vi "PH_IEEE1394Camera.get Cam Attributes.vi"(0 "i ref in":refnum<vi>, 2 "IMAQ1394 Session In":T1, 4 "Cam Error in":errorcluster, 5 "error in (no error)":errorcluster) -> (14 "i ref out":refnum<vi>, 16 "IMAQ1394 Session Out":T1, 18 "Cam Error out":errorcluster, 19 "error out":errorcluster)   [LabVIEW 2014, in "PH_IEEE1394Camera.lvlib"]
doc: "This VI gets the cam attributes and sets them to the GUI element."
uses:
  PH_IEEE1394Camera.lvlib
  <vilib>/userdefined/High Color/IMAQdx.ctl
  <vilib>/vision/driver/NI_Vision_Acquisition_Software.lvlib
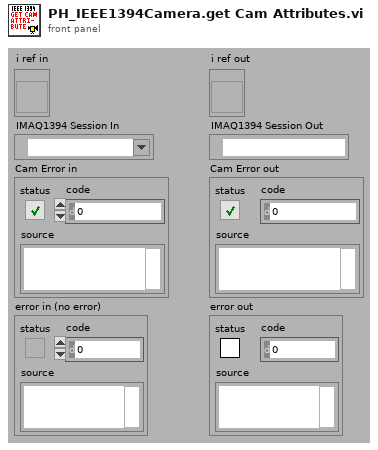
[diagram p1: front panel]
types:
  T1 = typedef "IMAQdx.ctl" = refnum<k21>
  T2 = typedef "PH_IEEE1394Camera.lvlib/PH_IEEE1394Camera.i attribute.ctl" = cluster{"Gui Refs":cluster{"Brightness":refnum<vi>, "Shutter":refnum<vi>, "Gain":refnum<vi>, "Center of Gravity":refnum<vi>, "Supported Video Modes":refnum<vi>, "Trigger Polarity":refnum<vi>, "Trigger Mode":refnum<vi>, "Trigger Timeout":refnum<vi>, "Bit Depth":refnum<vi>, "Video Mode":refnum<vi>, "Top":refnum<vi>, "Bottom":refnum<vi>, "Left":refnum<vi>, "Right":refnum<vi>, "Set ROI to Maximum":refnum<vi>, "Camera Details":refnum<vi>, "Current Cam Attributes":refnum<vi>, "Attribute to set":refnum<vi>, "Num Value":refnum<vi>, "String Value":refnum<vi>, "Bool Value":refnum<vi>, "Set Cam Attribute":refnum<vi>}, "Cam":cluster{"IMAQ1394 Session":T1, "Camera Details":T3}, "Current Attributes":T4[], "Supported Video Modes ":cluster{"Video Mode":u32, "Video Mode Name":string}[], "Wanted Attributes":cluster{"Name":string, "Num Value":dbl, "String Value":string, "Boolean Value":bool}[], "Cam Attributes":T6}
  T3 = typedef "PH_IEEE1394Camera.lvlib/PH_IEEE1394Camera.Cam Details.ctl" = cluster{"Model":string, "Serial Number":dbl, "Cam name (Machinery)":string, "Bus Type":string}
  T4 = typedef "PH_IEEE1394Camera.lvlib/PH_IEEE1394Camera.Cam Attribute.ctl" = cluster{"Information":cluster{"Type":T5, "Readable":bool, "Writable":bool, "Name":string}, "Num Value":dbl, "String Value":string, "Maximum":dbl, "Minimum":dbl, "Units":string, "Description":string, "EnumStrings[]":string[], "EnumValues[]":u32[], "Boolean Value":bool}
  T5 = typedef "NI_Vision_Acquisition_Software.lvlib/IMAQdx Attribute Type.ctl" = enum32{"U32", "I64", "DBL", "String", "Enum", "Bool", "Command"}
  T6 = typedef "PH_IEEE1394Camera.lvlib/PH_IEEE1394Camera.Relevant Cam Attributes.ctl" = cluster{"Video Mode":cluster{"Name":string, "Index":i32}, "Brightness":cluster{"Name":string, "Index":i32}, "Gain":cluster{"Name":string, "Index":i32}, "Shutter":cluster{"Name":string, "Index":i32}, "Trigger Pol":cluster{"Name":string, "Index":i32}, "Trigger Mode":cluster{"Name":string, "Index":i32}, "Timeout":cluster{"Name":string, "Index":i32}, "Bit Depth":cluster{"Name":string, "Index":i32}, "Pixel Bits":cluster{"Name":string, "Index":i32}, "Pixel Bytes":cluster{"Name":string, "Index":i32}, "Left":cluster{"Name":string, "Index":i32}, "Right":cluster{"Name":string, "Index":i32}, "Top":cluster{"Name":string, "Index":i32}, "Bottom":cluster{"Name":string, "Index":i32}}
  T7 = cluster{"Name":string, "Num Value":dbl, "String Value":string, "Boolean Value":bool}
  T8 = cluster{"Attribute Type":T5, "Readable":bool, "Writable":bool, "Attribute Name":string}[]
  T9 = cluster{"[0]":cluster{"Name":string, "Index":i32}, "[1]":cluster{"Name":string, "Index":i32}, "[2]":cluster{"Name":string, "Index":i32}, "[3]":cluster{"Name":string, "Index":i32}, "[4]":cluster{"Name":string, "Index":i32}, "[5]":cluster{"Name":string, "Index":i32}, "[6]":cluster{"Name":string, "Index":i32}, "[7]":cluster{"Name":string, "Index":i32}, "[8]":cluster{"Name":string, "Index":i32}, "[9]":cluster{"Name":string, "Index":i32}, "[10]":cluster{"Name":string, "Index":i32}, "[11]":cluster{"Name":string, "Index":i32}, "[12]":cluster{"Name":string, "Index":i32}, "[13]":cluster{"Name":string, "Index":i32}}
  T10 = cluster{"Name":string, "Num Value":dbl, "String Value":string, "Boolean Value":bool}[]
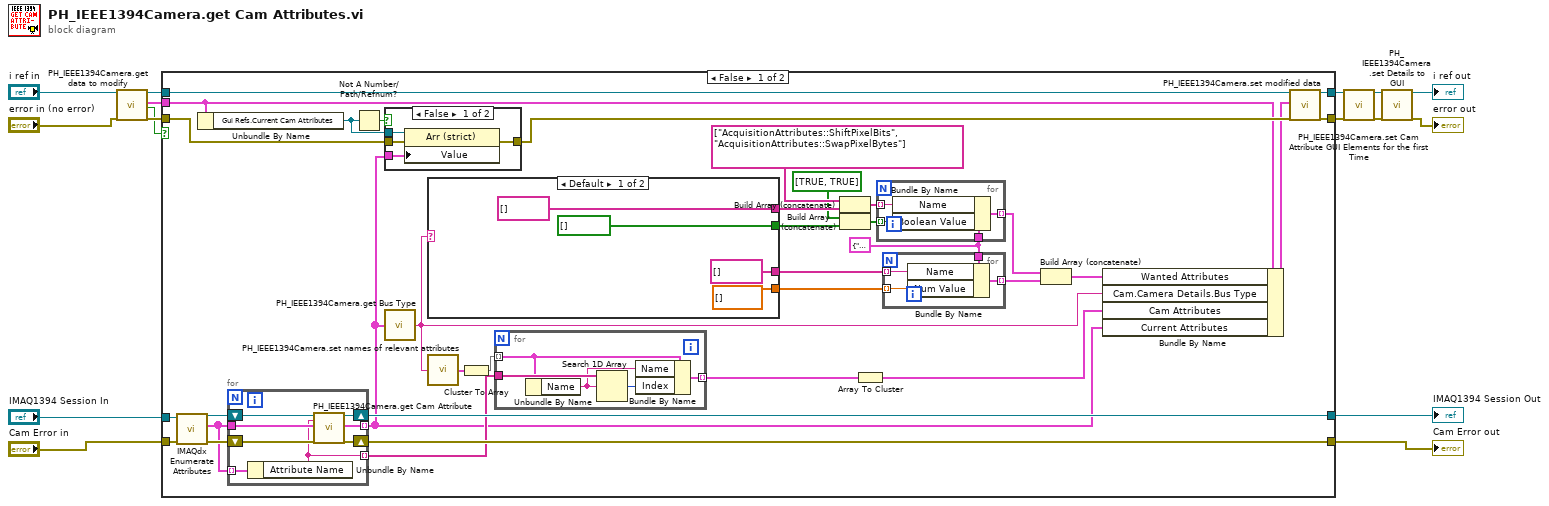
[diagram p0: block diagram]
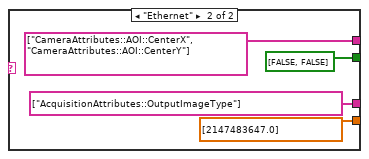
[diagram p2: hidden frame]
diagram:
  n1 = call "PH_IEEE1394Camera.get data to modify.vi"("i ref in"="i ref in", "error in (no error)"="error in (no error)") -> ("i ref out"=w13:refnum<vi>, "i attribute"=w16:T2, "timed out"=w12:bool, "error out"=w14:errorcluster)  [unwired: 14 in]
  n2 = case shown="False" w12 {
    tunnel: w16 -> [w44 _]
    tunnel: w14 -> [w49 w89]
    tunnel: w13 -> [w48 w88]
    tunnel: [w47 w88] -> w6
    tunnel: [w34 w89] -> w5
    tunnel: [w43 w87] -> w10
    tunnel: [w42 w86] -> w9
    tunnel: "IMAQ1394 Session In" -> [w33 w87]
    tunnel: "Cam Error in" -> [w32 w86]
    frame False {
      w20 = T7 {"Name"="", "Num Value"=0.0, "String Value"="", "Boolean Value"=FALSE} ("Attribute")
      n3 = call <vilib>:"IMAQdx Enumerate Attributes.vi"("error in"=w32, "Session In"=w33) -> ("error out"=w41:errorcluster, "Attribute Information Array"=w39:T8, "Session Out"=w40:T1)  [unwired: 7 in]
      n4 = Unbundle By Name(w44) -> ("Gui Refs.Current Cam Attributes"=w50:refnum<vi>)
      n5 = for {
        tunnel: w39 -> [w79] mode=indexing
        tunnel: w39 -> [w80]
        tunnel: [w78] -> w27 mode=indexing
        shift-right: [w76] -> w43
        shift-left: w40 -> [w75]
        shift-right: [w77] -> w42
        shift-left: w41 -> [w74]
        tunnel: [w73] -> w38 mode=indexing
        n6 = Unbundle By Name(w79) -> ("Attribute Name"=w73:string)
        n7 = call "PH_IEEE1394Camera.get Cam Attribute.vi"("IMAQ1394 Session In"=w75, "Cam Attribute Name"=w73, "Attribute Information Array"=w80, "Cam Error in"=w74) -> ("IMAQ1394 Session Out"=w76:T1, "Cam Attribute Value"=w78:T4, "Cam Error out"=w77:errorcluster)  [unwired: 12 in, 1 out]
      }
      n8 = Not A Number/Path/Refnum?(number/path/refnum=w50) -> (NaN/Path/Refnum?=w51:bool)
      n9 = case shown="False" w51 {
        tunnel: w50 -> [w84 _]
        tunnel: [w83 w85] -> w46
        tunnel: w49 -> [w82 w85]
        tunnel: w27 -> [w81 _]
        frame False {
          n10 = property class="Arr (strict)"(reference=w84, error in=w82, "Value"=w81) -> (error out=w83:errorcluster)  [unwired: 1 out]
        }
        frame True {
        }
      }
      n11 = call "PH_IEEE1394Camera.get Bus Type.vi"("Camera Attributes"=w27) -> ("Bus Type"=w26:string)
      n12 = case shown="Default" w26 {
        tunnel: [string[] [] string[] ["CameraAttributes::AOI::CenterX", "CameraAttributes::AOI::CenterY"]] -> w28
        tunnel: [bool[] [] bool[] [FALSE, FALSE]] -> w23
        tunnel: [string[] [] string[] ["AcquisitionAttributes::OutputImageType"]] -> w18
        tunnel: [dbl[] [] dbl[] [2147483647.0]] -> w17
        frame Default {
        }
        frame "Ethernet" {
        }
      }
      n13 = call "PH_IEEE1394Camera.set names of relevant attributes.vi"("Bus Type"=w26) -> ("Relevant Cam Attributes"=w31:T6)
      n14 = Cluster To Array(cluster=w31) -> (array=w36:cluster{"Name":string, "Index":i32}[])
      n15 = for {
        tunnel: w38 -> [w72]
        tunnel: w36 -> [w71] mode=indexing
        tunnel: [w69] -> w35 mode=indexing
        n16 = Unbundle By Name(w71) -> ("Name"=w70:string)
        n17 = Search 1D Array(1D array=w72, element=w70) -> (index of element=w68:i32)  [unwired: 1 in]
        n18 = Bundle By Name(cluster=w71, "Name"=w70, "Index"=w68) -> (w69:cluster{"Name":string, "Index":i32})
      }
      n19 = Build Array (concatenate)(string[] ["AcquisitionAttributes::ShiftPixelBits", "AcquisitionAttributes::SwapPixelBytes"], w28) -> (w29:string[])
      n20 = Build Array (concatenate)(bool[] [TRUE, TRUE], w23) -> (w25:bool[])
      n21 = Array To Cluster(array=w35) -> (cluster=w37:T9)
      n22 = for {
        tunnel: w20 -> [w67]
        tunnel: [w66] -> w21 mode=indexing
        tunnel: w25 -> [w65] mode=indexing
        tunnel: w29 -> [w64] mode=indexing
        n23 = Bundle By Name(cluster=w67, "Name"=w64, "Boolean Value"=w65) -> (w66:T7)
      }
      n24 = for {
        tunnel: w20 -> [w55]
        tunnel: [w54] -> w19 mode=indexing
        tunnel: w18 -> [w53] mode=indexing
        tunnel: w17 -> [w52] mode=indexing
        n25 = Bundle By Name(cluster=w55, "Name"=w53, "Num Value"=w52) -> (w54:T7)
      }
      n26 = Build Array (concatenate)(w21, w19) -> (w22:T10)
      n27 = Bundle By Name(cluster=w44, "Wanted Attributes"=w22, "Cam.Camera Details.Bus Type"=w26, "Cam Attributes"=w37, "Current Attributes"=w27) -> (w45:T2)
      n28 = call "PH_IEEE1394Camera.set modified data.vi"("i ref in"=w48, "i attribute"=w45, "error in (no error)"=w46) -> ("i ref out"=w47:refnum<vi>, "error out"=w34:errorcluster)  [unwired: 15 in]
    }
    frame True {
    }
  }
  "IMAQ1394 Session Out" <- w10
  "Cam Error out" <- w9
  n29 = call "PH_IEEE1394Camera.set Cam Attribute GUI Elements for the first Time.vi"("i ref in"=w6, "error in (no error)"=w5) -> ("i ref out"=w4:refnum<vi>, "error out"=w2:errorcluster)  [unwired: 16 in]
  n30 = call "PH_IEEE1394Camera.set Details to GUI.vi"("VI in"=w4, "error in (no error)"=w2) -> ("VI out"=→"i ref out":refnum<vi>, "error out"=→"error out":errorcluster)  [unwired: 16 in]
